vi "LEBITplc.ReadDbase.vi"(0 "i ref in":refnum<vi>, 2 "Data Source":string="LBADD", 5 "error in (no error)":errorcluster, 9 "Associated Panels":string[](array[string])=["buncher", "testionsource", "penning", "buntopenning", "penningeject", "mcp&phosvol", "gascell", "ionguide", "n4tobob1", "bob1tobun", "deceltobun", "las"]) -> (14 "i ref out":refnum<vi>, 15 "ListOfBases":string[](array[string]), 16 "DBArray":string[][](array[string]), 17 "Min&MaxArray":string[][](array[string]), 18 "Scale And Offset Array":string[][](array[string]), 19 "error out":errorcluster)   [LabVIEW 2014, in "LEBITplc.lvlib"]
uses:
  LEBITplc.lvlib
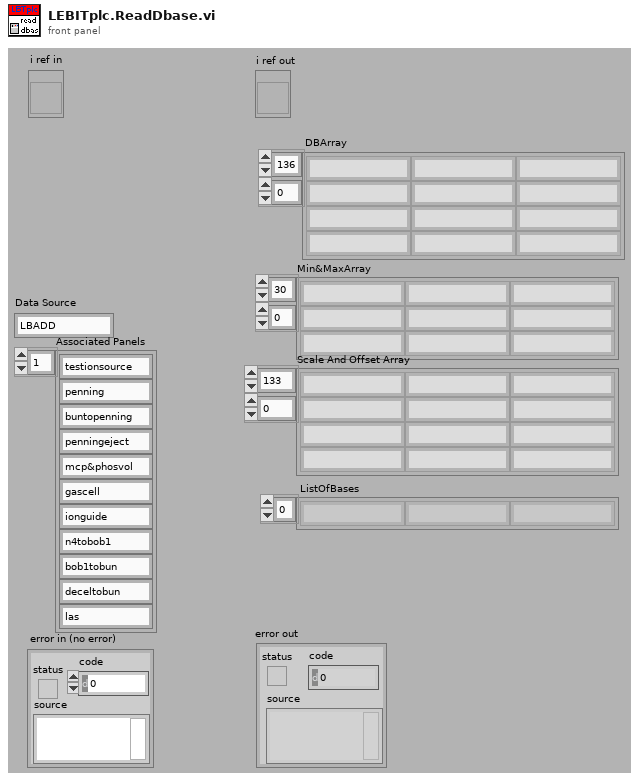
[diagram p1: front panel]
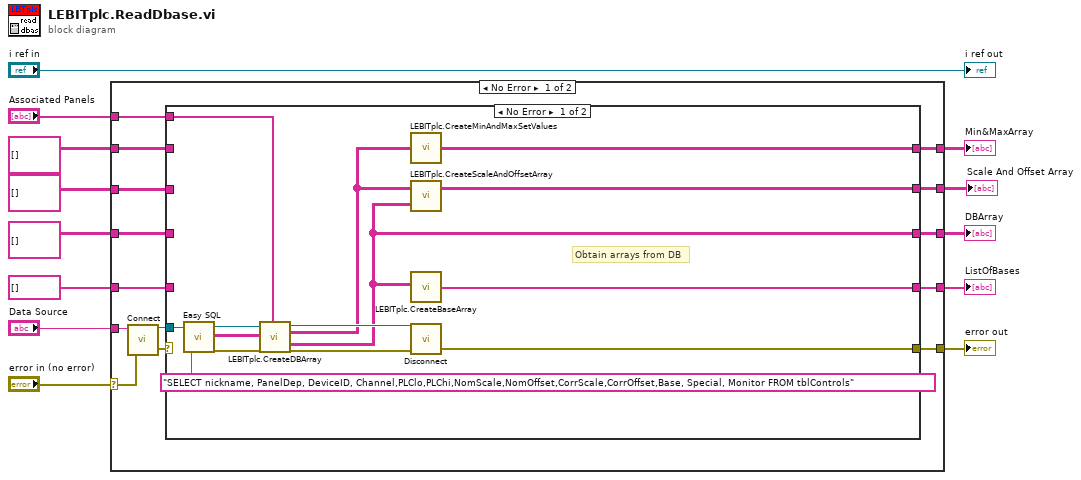
[diagram p0: block diagram]
diagram:
  n1 = case shown="No Error" "error in (no error)" {
    selector: "error in (no error)" -> [w26 w51]
    tunnel: "Data Source" -> [w27 _]
    tunnel: [w23 w51] -> w9
    tunnel: string[][] [] ("DBArrayIn") -> [w22 w50]
    tunnel: [w21 w50] -> w11
    tunnel: [w20 w49] -> w6
    tunnel: string[][] [] ("DBArrayIn") -> [w19 w49]
    tunnel: [w18 w48] -> w4
    tunnel: string[] [] ("DBArrayIn") -> [w17 w48]
    tunnel: string[][] [] ("DBArrayIn") -> [w16 w47]
    tunnel: [w15 w47] -> w2
    tunnel: "Associated Panels" -> [w14 _]
    frame No Error {
      n2 = call <vilib>:"Connect.vi"("error in (no error)"=w26, "data source name"=w27) -> ("error out"=w24:errorcluster, "Connection"=w25:refnum<k7>)  [unwired: 2 in]
      n3 = case shown="No Error" w24 {
        selector: w24 -> [_ w46]
        tunnel: w25 -> [w32 _]
        tunnel: [w36 w46] -> w23
        tunnel: w22 -> [_ w45]
        tunnel: [w31 w45] -> w21
        tunnel: [w34 w44] -> w20
        tunnel: w19 -> [_ w44]
        tunnel: [w35 w43] -> w18
        tunnel: w17 -> [_ w43]
        tunnel: w16 -> [_ w42]
        tunnel: [w33 w42] -> w15
        tunnel: w14 -> [w28 _]
        frame No Error {
          # "Obtain arrays from DB"
          n4 = call <vilib>:"Easy SQL.vi"("connection"=w32, "SQL statement"="SELECT nickname, PanelDep, DeviceID, Channel,PLClo,PLChi,NomScale,NomOffset,CorrScale,CorrOffset,Base, Special, Monitor FROM tblControls") -> ("connection"=w37:refnum<k7>, "error out"=w39:errorcluster, "query results"=w30:string[][])  [unwired: 1 in, 2 out]
          n5 = call "LEBITplc.CreateDBArray.vi"("connection in"=w37, "query results"=w30, "error in"=w39, "Associated Panels"=w28) -> ("connection out"=w40:refnum<k7>, "InfoArray"=w29:string[][], "DBArray"=w31:string[][], "error out"=w38:errorcluster)  [unwired: 12 in]
          n6 = call "LEBITplc.CreateMinAndMaxSetValues.vi"("Info Array from DB"=w29) -> ("Min & Max Array"=w34:string[][])
          n7 = call "LEBITplc.CreateScaleAndOffsetArray.vi"("DBArray"=w31, "Info Array from DB"=w29) -> ("Scale And Offset Array"=w33:string[][])  [unwired: 1 in]
          n8 = call "LEBITplc.CreateBaseArray.vi"("DBArray"=w31) -> ("ListOfBases"=w35:string[])  [unwired: 4 in]
          n9 = call <vilib>:"Disconnect.vi"("error in (no error)"=w38, "connection"=w40) -> ("error out"=w36:errorcluster)  [unwired: 1 in]
        }
        frame Error {
        }
      }
    }
    frame Error {
      (unwired) 0
    }
  }
  "error out" <- w9
  "DBArray" <- w11
  "Min&MaxArray" <- w6
  "ListOfBases" <- w4
  "Scale And Offset Array" <- w2
  "i ref out" <- "i ref in"
